vi "Set Menu.vi"(8 "error in (no error)":errorcluster, 10 "RTM Data in":refnum<class "Menu Data.lvclass">, 11 "ProjectData in":refnum<class "Project Data.lvclass">) -> (0 "error out":errorcluster, 2 "Replaced?":bool, 3 "ProjectData out":refnum<class "Project Data.lvclass">)   [LabVIEW 2013, in "SET Project Data.lvlib" / "Project Data.lvclass"]
uses:
  Project Data.lvclass
  Menu Class/Menu Data.lvclass
  Menu Class/Menu Data.lvclass/Menu Data.ctl
  Project Data.lvclass/Project Data.ctl
  Menu Class/Read Menu Path (Relative).vi
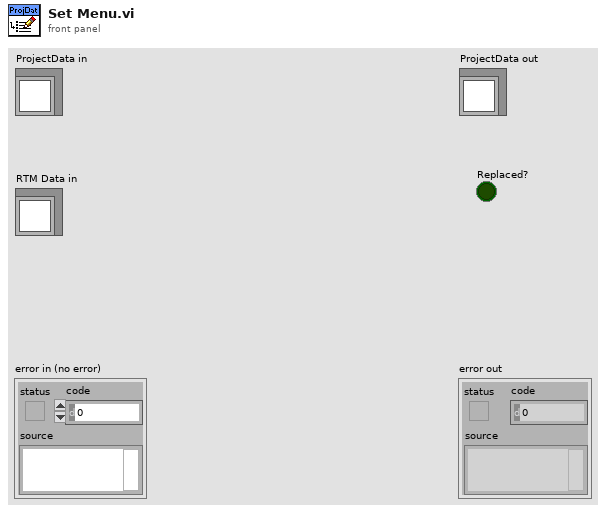
[diagram p1: front panel]
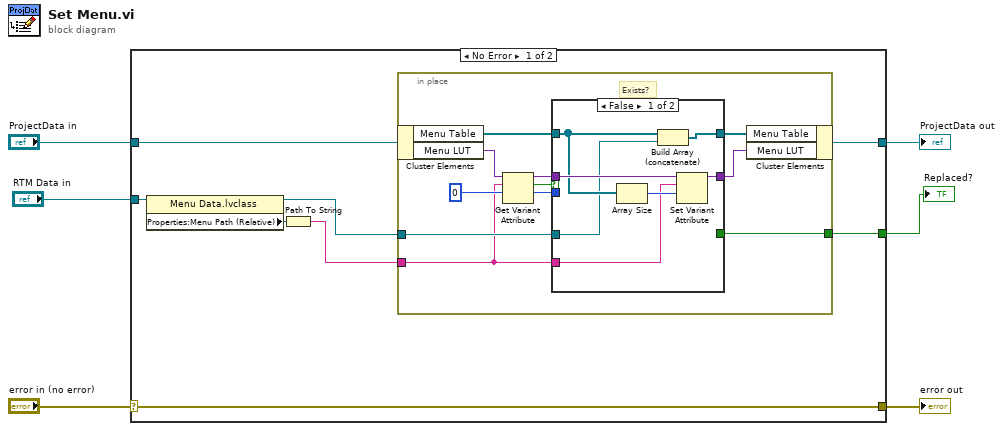
[diagram p0: block diagram]
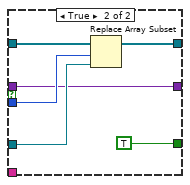
[diagram p2: hidden frame]
diagram:
  n1 = case shown="No Error" "error in (no error)" {
    selector: "error in (no error)" -> [w14 w40]
    tunnel: [w14 w40] -> w5
    tunnel: [w10 w39] -> w3
    tunnel: "ProjectData in" -> [w11 w39]
    tunnel: "RTM Data in" -> [w13 _]
    tunnel: [w7 _] -> w1
    frame No Error {
      n2 = property class="Menu Data.lvclass"(reference=w13) -> (reference out=w9:refnum<class "Menu Data.lvclass">, "Properties:Menu Path (Relative)"=w12:path)  [unwired: 1 in, 1 out]
      n3 = Path To String(path=w12) -> (string=w8:string)
      n4 = in-place {
        in-place-border: w9 -> [w23]
        in-place-border: w8 -> [w16]
        in-place-border: [w15] -> w7
        # "Exists?"
        n5 = in-place-cluster #1(w11) -> ("Menu Table"=w25:refnum<class "Menu Data.lvclass">[], "Menu LUT"=w22:variant)
        n6 = Get Variant Attribute(Variant=w22, name=w16, default value (empty Variant)=0) -> (duplicate Variant=w18:variant, found=w21:bool, value=w19:i32)  [unwired: 1 in, 1 out]
        n7 = case shown="False" w21 {
          tunnel: w25 -> [w28 w38]
          tunnel: [w26 w37] -> w24
          tunnel: w23 -> [w27 w36]
          tunnel: w19 -> [_ w35]
          tunnel: w18 -> [w31 w34]
          tunnel: [w32 w34] -> w17
          tunnel: w16 -> [w29 _]
          tunnel: [_ TRUE] -> w15
          frame False {
            n8 = Array Size(array=w28) -> (size(s)=w30:i32)
            n9 = Build Array (concatenate)(w28, w27) -> (w26:refnum<class "Menu Data.lvclass">[])
            n10 = Set Variant Attribute(Variant=w31, name=w29, value=w30) -> (Variant out=w32:variant)  [unwired: 1 in, 2 out]
          }
          frame True {
            n11 = Replace Array Subset(array=w38, new element=w36, index=w35) -> (w37:refnum<class "Menu Data.lvclass">[])
          }
        }
        n12 = in-place-cluster #1("Menu Table"=w24, "Menu LUT"=w17) -> (w10:refnum<class "Project Data.lvclass">)
      }
    }
    frame Error {
    }
  }
  "error out" <- w5
  "ProjectData out" <- w3
  "Replaced?" <- w1
